vi "Image_2d u32 to 3d u8.vi"(0 "Image_2d_u32":u32[][](array[numeric]) format="%08x", 5 "error in (no error)":errorcluster) -> (14 "Image_3d_u8":u8[][][](array[numeric]) format="%0d", 19 "error out":errorcluster)   [LabVIEW 2016]
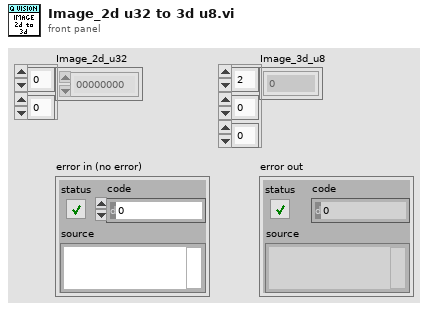
[diagram p1: front panel]
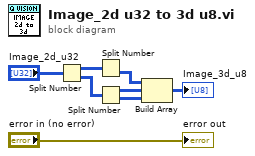
[diagram p0: block diagram]
diagram:
  n1 = Split Number(x="Image_2d_u32") -> (hi(x)=w3:u16[][], lo(x)=w4:u16[][])
  n2 = Split Number(x=w3) -> (lo(x)=w5:u8[][])  [unwired: 1 out]
  n3 = Split Number(x=w4) -> (hi(x)=w6:u8[][], lo(x)=w7:u8[][])
  n4 = Build Array(w5, w6, w7) -> (→"Image_3d_u8":u8[][][])
  "error out" <- "error in (no error)"
